vi "Stopwatch - Solution.vi"() -> ()   [LabVIEW 2014]
panel:
  out "Numeric":dbl format="%<%M:%S%2u>t"
  in  "Reset":bool
  in  "Stop":bool
  in  "Start":bool
  out "Time":dbl(knob) scale=0.0..60.0 scale format="%#.2f"
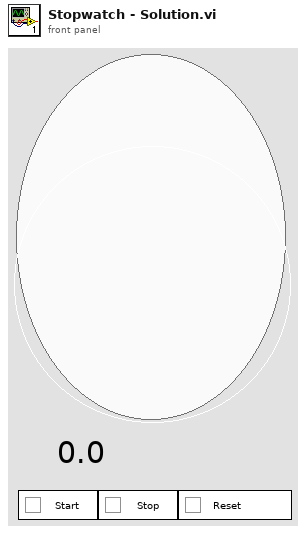
[diagram p1: front panel]
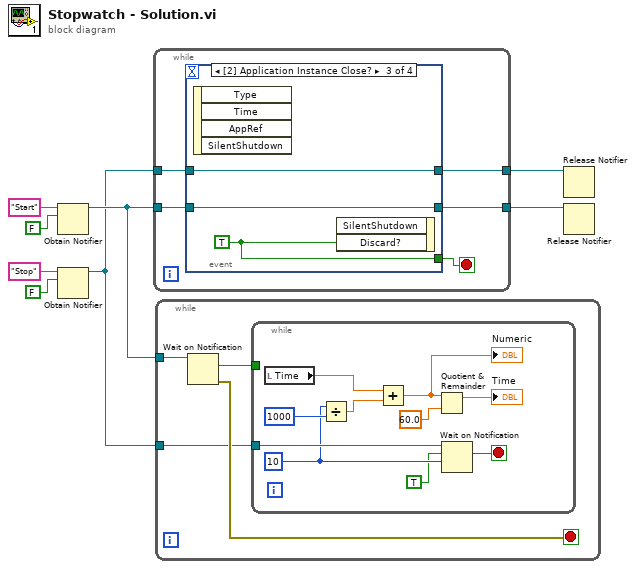
[diagram p0: block diagram]
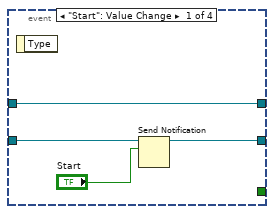
[diagram p2: hidden frame]
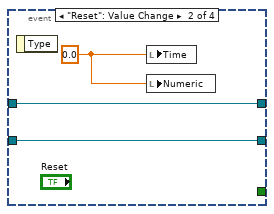
[diagram p3: hidden frame]
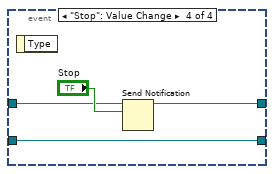
[diagram p4: hidden frame]
diagram:
  n1 = Obtain Notifier(name (unnamed)="Start", notification data type=FALSE ("Start")) -> (notifier out=w4:refnum<notifier>)  [unwired: 2 in, 2 out]
  n2 = Obtain Notifier(name (unnamed)="Stop", notification data type=FALSE ("Start")) -> (notifier out=w3:refnum<notifier>)  [unwired: 2 in, 2 out]
  n3 = while {
    tunnel: w4 -> [w13]
    tunnel: w3 -> [w11]
    tunnel: [w10] -> w2
    tunnel: [w9] -> w1
    stop <- w12 stop-if-true
    n4 = event shown="[2] Application Instance Close?" {
      selector: _ -> [_ _ _ _]
      dyn-events: _ -> [_ _ _ _]
      timeout: _ -> [_ _ _ _]
      tunnel: w13 -> [w17 w20 w22 w24]
      tunnel: [_ _ w23 _] -> w12
      tunnel: w11 -> [w14 w19 w21 w26]
      tunnel: [w15 w20 w22 w24] -> w10
      tunnel: [w14 w19 w21 w25] -> w9
      event "Start": Value Change {
        n5 = event-data() -> ()  [unwired: 1 in, 1 out]
        n6 = Send Notification(notification="Start", notifier=w17) -> (notifier out=w15:refnum<notifier>)  [unwired: 1 in, 1 out]
      }
      event "Reset": Value Change {
        w18 = 0.0 ("Time")
        n7 = event-data() -> ()  [unwired: 1 in, 1 out]
        n8 = local write "Time"(w18) -> ()
        n9 = local write "Numeric"(w18) -> ()
      }
      event Application Instance Close? {
        w23 = TRUE ("Discard?")
        n10 = event-data() -> ()  [unwired: 1 in, 4 out]
        n11 = event-data("Discard?"=w23) -> ()  [unwired: 2 in, 1 out]
      }
      event "Stop": Value Change {
        n12 = event-data() -> ()  [unwired: 1 in, 1 out]
        n13 = Send Notification(notification="Stop", notifier=w26) -> (notifier out=w25:refnum<notifier>)  [unwired: 1 in, 1 out]
      }
    }
  }
  n14 = while {
    tunnel: w4 -> [w31]
    tunnel: w3 -> [w29]
    stop <- w30 stop-if-true
    n15 = Wait on Notification(notifier=w31) -> (notification=w28:bool, error out=w30:errorcluster)  [unwired: 3 in, 2 out]
    n16 = while {
      tunnel: w29 -> [w41]
      tunnel: w28 -> [_]
      stop <- w40 stop-if-true
      w38 = 10 ("timeout in ms (-1)")
      n17 = local read "Time"() -> (w35:dbl)
      n18 = Divide(x=w38, y=1000 ("timeout in ms (-1)")) -> (x/y=w37:dbl)
      n19 = Add(x=w35, y=w37) -> (x+y=w32:dbl)
      "Numeric" <- w32
      n20 = Quotient & Remainder(x=w32, y=60.0) -> (x-y*floor(x/y)=→"Time":dbl)  [unwired: 1 out]
      n21 = Wait on Notification(notifier=w41, ignore previous (F)=TRUE, timeout in ms (-1)=w38) -> (notification=w40:bool)  [unwired: 1 in, 3 out]
    }
  }
  n22 = Release Notifier(notifier=w1) -> ()  [unwired: 2 in, 3 out]
  n23 = Release Notifier(notifier=w2) -> ()  [unwired: 2 in, 3 out]
